vi "TL midbrain ACT.vi"(3 "error in":errorcluster, 4 "Behavior\nVelocity":dbl=20.0, 5 "Behavior arrays":T1, 6 "Forebrain ACT":dbl[](array[numeric])) -> (0 "error out":errorcluster, 1 "Act Com":T2, 2 "Waveform Graph":cluster{dbl, dbl, dbl[]}(graph))   [LabVIEW 2014]
doc: "This vi is the midbrain ACT routine."
panel:
  out "Max value":dbl
  out "Peak Heading":dbl
  out "Desired\nSpeed":dbl format="%#_13g"
  out "Desired \nRudder":dbl format="%#_13g"
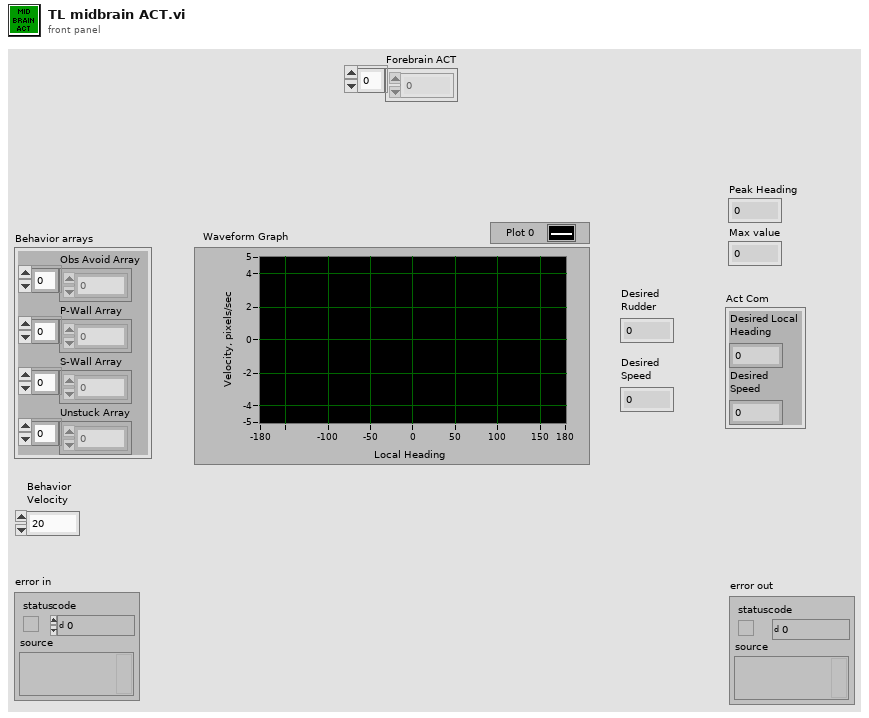
[diagram p1: front panel]
types:
  T1 = cluster{"Obs Avoid Array":dbl[], "P-Wall Array":dbl[], "S-Wall Array":dbl[], "Unstuck Array":dbl[]}
  T2 = cluster{"Desired Local\nHeading":dbl, "Desired\nSpeed":dbl}
  T3 = cluster{"Peak Heading":dbl, "Behavior\nVelocity":dbl}
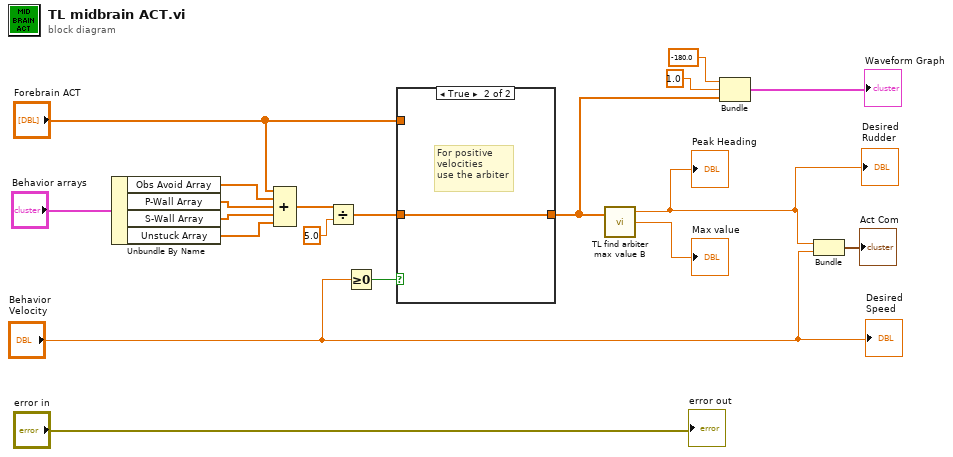
[diagram p0: block diagram]
diagram:
  n1 = Unbundle By Name("Behavior arrays") -> ("Obs Avoid Array"=w17:dbl[], "P-Wall Array"=w16:dbl[], "S-Wall Array"=w15:dbl[], "Unstuck Array"=w14:dbl[])
  n2 = Compound Arithmetic op=ADD("Forebrain ACT", w17, w16, w15, w14) -> (w13:dbl[])
  n3 = Divide(x=w13, y=5.0) -> (x/y=w3:dbl[])
  n4 = Greater Or Equal To 0?(x="Behavior\nVelocity") -> (x >= 0?=w5:bool)
  n5 = case shown="True" w5 {
    tunnel: w3 -> [_ w21]
    tunnel: [w20 w21] -> w2
    tunnel: "Forebrain ACT" -> [w20 _]
    frame False {
      # "If velocity is negative\ndo use the arbiter\njust the Forebrain"
    }
    frame True {
      # "For positive \nvelocities\nuse the arbiter"
    }
  }
  n6 = call "TL find arbiter max value B.vi"("ACT array"=w2) -> ("Peak Heading"=w6:dbl, "Max value"=→"Max value":dbl)  [unwired: 1 in, 1 out]
  "Desired \nRudder" <- w6
  "Peak Heading" <- w6
  n7 = Bundle(-180.0, 1.0, "Forebrain ACT"=w2) -> (→"Waveform Graph":cluster{dbl, dbl, "Forebrain ACT":dbl[]})  [unwired: 1 in]
  n8 = Bundle("Peak Heading"=w6, "Behavior\nVelocity"="Behavior\nVelocity") -> (→"Act Com":T3)  [unwired: 1 in]
  "Desired\nSpeed" <- "Behavior\nVelocity"
  "error out" <- "error in"
